vi "InstantiateAccessorVIs.vi"(7 "Include error terminals":bool, 8 "error in (no error)":errorcluster, 11 "BaseAccessorScripter in":refnum<class "BaseAccessorScripter.lvclass">) -> (0 "error out":errorcluster, 3 "BaseAccessorScripter out":refnum<class "BaseAccessorScripter.lvclass">)   [LabVIEW 2021, in "MemberVICreation.lvlib" / "BaseAccessorScripter.lvclass"]
uses:
  <resource>/Framework/Providers/LVClassLibrary/NewAccessors/BaseAccessorScripter/BaseAccessorScripter.lvclass
  <resource>/Framework/Providers/LVClassLibrary/NewAccessors/BaseAccessorScripter/BaseAccessorScripter.lvclass/BaseAccessorScripter.ctl
  <resource>/Framework/Providers/LVClassLibrary/NewAccessors/MemberVICreation.lvlib
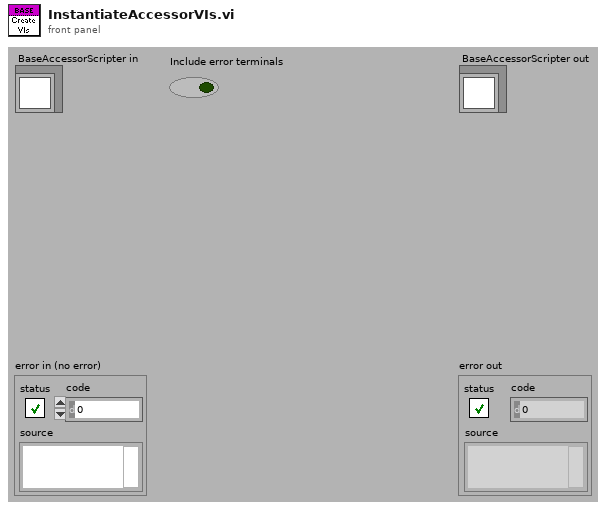
[diagram p1: front panel]
types:
  T1 = enum32{"invalid VI type", "Standard VI", "Control VI", "Global VI", "Polymorphic VI", "Configuration VI", "SubSystem", "Facade VI", "Method VI"}
  T2 = typedef "MemberVICreation.lvlib/CLSUIP_Access.ctl" = enum16{"Read", "Write", "R/W"}
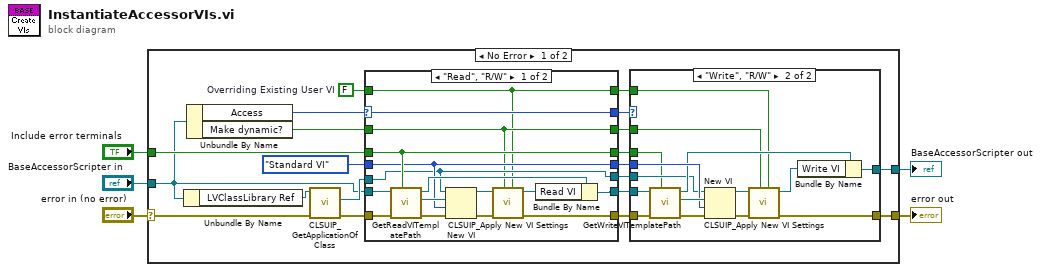
[diagram p0: block diagram]
diagram:
  n1 = case shown="No Error" "error in (no error)" {
    selector: "error in (no error)" -> [w24 w68]
    tunnel: [w20 w68] -> w4
    tunnel: [w19 w67] -> w2
    tunnel: "BaseAccessorScripter in" -> [w11 w67]
    tunnel: "Include error terminals" -> [w17 _]
    frame No Error {
      w7 = FALSE  # Overriding Existing User VI
      n2 = Unbundle By Name(w11) -> ("LVClassLibrary Ref"=w25:refnum<vi>)
      n3 = Unbundle By Name(w11) -> ("Access"=w10:T2, "Make dynamic?"=w9:bool)
      n4 = call <resource>:"CLSUIP_GetApplicationOfClass.vi"("error in (no error)"=w24, "LVClassLibrary Ref"=w25) -> ("error out"=w23:errorcluster, "Application"=w13:refnum<vi>)  [unwired: 8 out]
      n5 = case shown="\"Read\", \"R/W\"" w10 {
        selector: w10 -> [w52 w64]
        tunnel: w11 -> [w58 w66]
        tunnel: w23 -> [w57 w65]
        tunnel: T1."Standard VI" ("vi type (standard vi)") -> [w50 w62]
        tunnel: [w46 w65] -> w21
        tunnel: [w53 w66] -> w22
        tunnel: w13 -> [w49 w61]
        tunnel: w17 -> [w51 w63]
        tunnel: [w52 w64] -> w16
        tunnel: [w51 w63] -> w15
        tunnel: [w50 w62] -> w14
        tunnel: [w49 w61] -> w12
        tunnel: w9 -> [w44 w60]
        tunnel: [w44 w60] -> w8
        tunnel: w7 -> [w43 w59]
        tunnel: [w43 w59] -> w6
        frame "Read", "R/W" {
          n6 = call-dynamic "GetReadVITemplatePath.vi"("Include error terminals"=w51, "error in (no error)"=w57, "BaseAccessorScripter in"=w58) -> ("error out"=w55:errorcluster, "VI Path"=w56:path, "BaseAccessorScripter out"=w54:refnum<class "BaseAccessorScripter.lvclass">)  [unwired: 6 out]
          n7 = New VI(8:w55, 9:w50, 10:w56, 11:w49) -> (0:w48:errorcluster, 3:w47:refnum<vi>)  [unwired: 3 out]
          n8 = call <resource>:"CLSUIP_Apply New VI Settings.vi"("Overriding Existing User VI"=w43, "Making dynamic?"=w44, "error in"=w48, "VI in"=w47) -> ("error out"=w46:errorcluster, "VI out"=w45:refnum<vi>)  [unwired: 6 in]
          n9 = Bundle By Name(cluster=w54, "Read VI"=w45) -> (w53:refnum<class "BaseAccessorScripter.lvclass">)
        }
        frame "Write" {
        }
      }
      n10 = case shown="\"Write\", \"R/W\"" w16 {
        tunnel: w22 -> [w27 w42]
        tunnel: w21 -> [w26 w41]
        tunnel: w14 -> [_ w38]
        tunnel: [w26 w30] -> w20
        tunnel: [w27 w36] -> w19
        tunnel: w12 -> [_ w35]
        tunnel: w15 -> [_ w34]
        tunnel: w8 -> [_ w29]
        tunnel: w6 -> [_ w28]
        frame "Read" {
        }
        frame "Write", "R/W" {
          n11 = call-dynamic "GetWriteVITemplatePath.vi"("Include error terminals"=w34, "error in (no error)"=w41, "BaseAccessorScripter in"=w42) -> ("error out"=w39:errorcluster, "VI Path"=w40:path, "BaseAccessorScripter out"=w37:refnum<class "BaseAccessorScripter.lvclass">)  [unwired: 6 out]
          n12 = New VI(8:w39, 9:w38, 10:w40, 11:w35) -> (0:w31:errorcluster, 3:w33:refnum<vi>)  [unwired: 3 out]
          n13 = call <resource>:"CLSUIP_Apply New VI Settings.vi"("Overriding Existing User VI"=w28, "Making dynamic?"=w29, "error in"=w31, "VI in"=w33) -> ("error out"=w30:errorcluster, "VI out"=w32:refnum<vi>)  [unwired: 6 in]
          n14 = Bundle By Name(cluster=w37, "Write VI"=w32) -> (w36:refnum<class "BaseAccessorScripter.lvclass">)
        }
      }
    }
    frame Error {
    }
  }
  "error out" <- w4
  "BaseAccessorScripter out" <- w2
